vi "Voltmetr_test.vi"() -> ()   [LabVIEW 2017]
uses:
  st_str Global.vi
  <vilib>/measure/maspectr.llb/FFT Spectrum (Mag-Phase) for N Chan.vi
  <vilib>/measure/NI_MAPro.lvlib
panel:
  in  "view":T1
  out "Waveform Graph 2":cluster{"f0":dbl, "df":dbl, "magnitude":dbl[]}[](graph)
  out "x > y?":bool
  out "Numeric":i32
  in  "Boolean":bool
  out "Waveform Graph":waveform(dbl)[](graph)
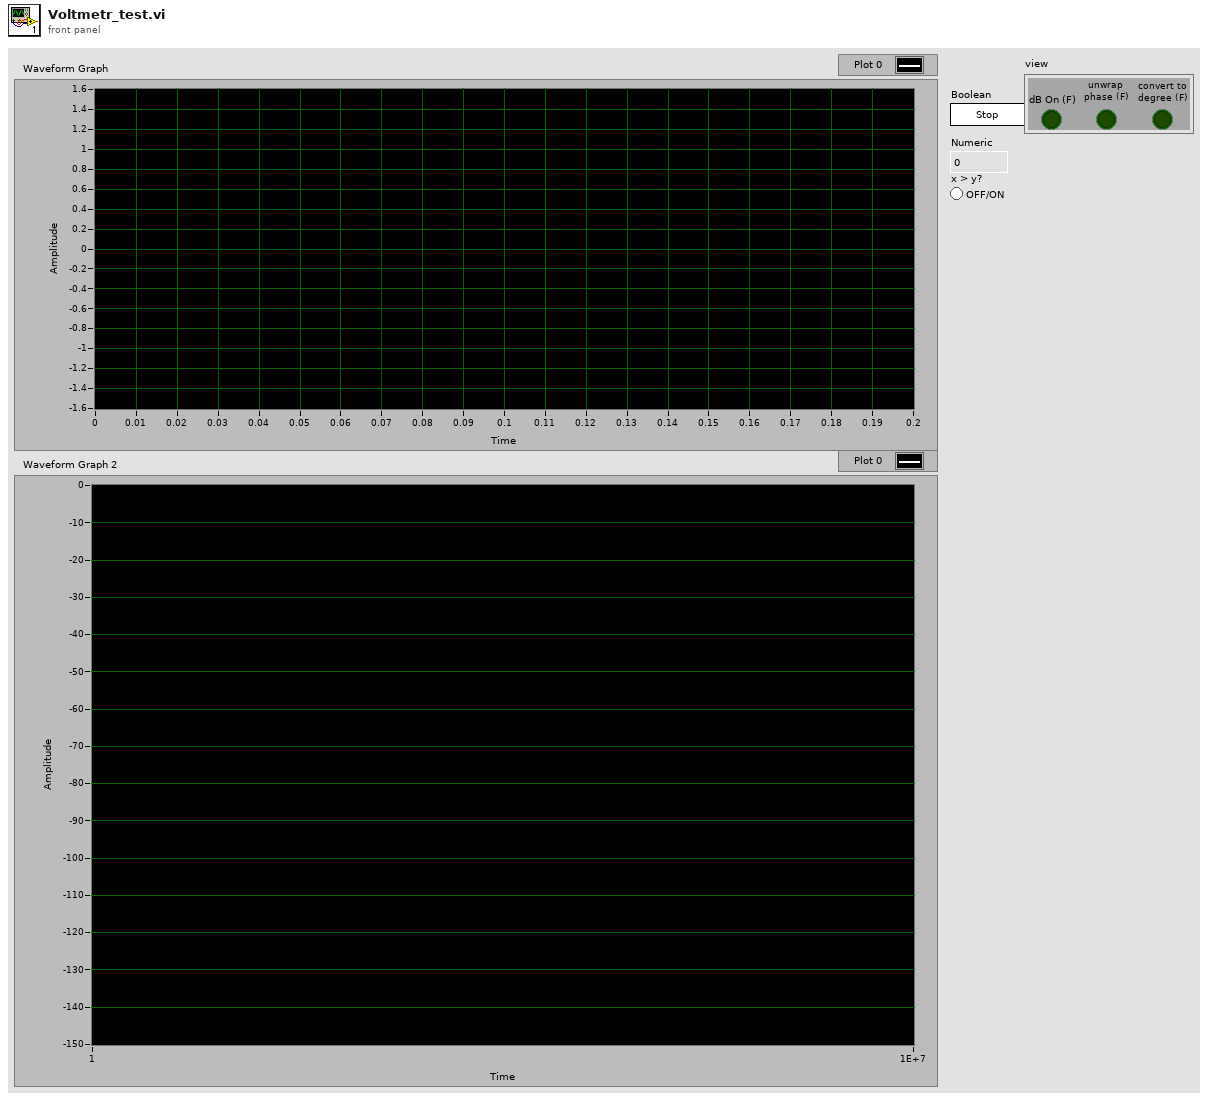
[diagram p1: front panel]
types:
  T1 = cluster{"dB On (F)":bool, "unwrap phase (F)":bool, "convert to degree (F)":bool}
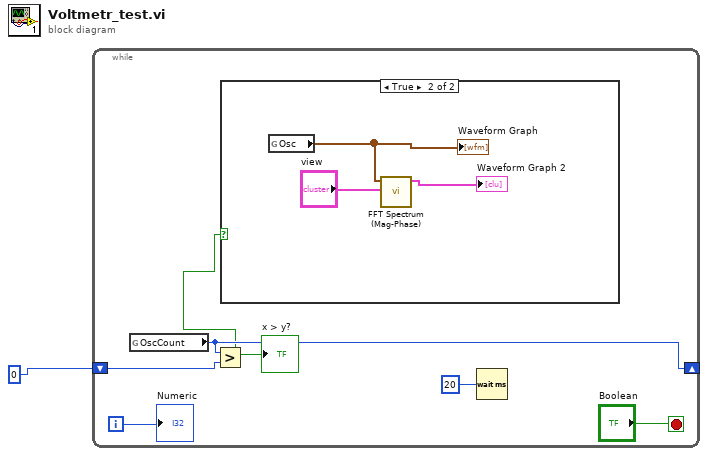
[diagram p0: block diagram]
diagram:
  n1 = while {
    shift-right: [w5] -> _
    shift-left: 0 ("OscCount") -> [w6]
    i -> [w3]
    stop <- "Boolean" stop-if-true
    n2 = global read "st_str Global.vi" "OscCount"() -> (w5:i32)
    n3 = Greater?(x=w5, y=w6) -> (0:w4:bool)
    "x > y?" <- w4
    n4 = case shown="True" w4 {
      frame False {
      }
      frame True {
        n5 = global read "st_str Global.vi" "Osc"() -> (w10:waveform(dbl)[])
        "Waveform Graph" <- w10
        n6 = call-poly <vilib>:"FFT Spectrum (Mag-Phase).vi"("view"="view", "time signals"=w10) -> ("magnitudes"=→"Waveform Graph 2":cluster{"f0":dbl, "df":dbl, "magnitude":dbl[]}[])  [unwired: 5 in, 4 out]
      }
    }
    n7 = Wait (ms)(milliseconds to wait=u32 20) -> ()  [unwired: 1 out]
    "Numeric" <- w3
  }
